vi "Drona Run Tests In Project.vi"   [LabVIEW 2016, in "Script.lvlib"]
uses:
  Script.lvlib
  <vilib>/Wiresmith Technology/G CLI/Argument Parser/Option Class/Option Configuration.ctl
  <vilib>/Wiresmith Technology/G CLI/Argument Parser/Option Class/Argument Type.ctl
  <vilib>/Wiresmith Technology/G CLI/Argument Parser/Option Class/Option.lvclass
  <vilib>/Wiresmith Technology/G CLI/Argument Parser/Option Set Class/Option Set.lvclass
types:
  T1 = typedef "Option Parser.lvlib/Option.lvclass/Option Configuration.ctl" = cluster{"Option Type":T2, "Option Labels":string[], "Key":string, "Description":string, "Required":bool, "Default Value":string}
  T2 = typedef "Option Parser.lvlib/Option.lvclass/Argument Type.ctl" = enum16{"flag", "value"}
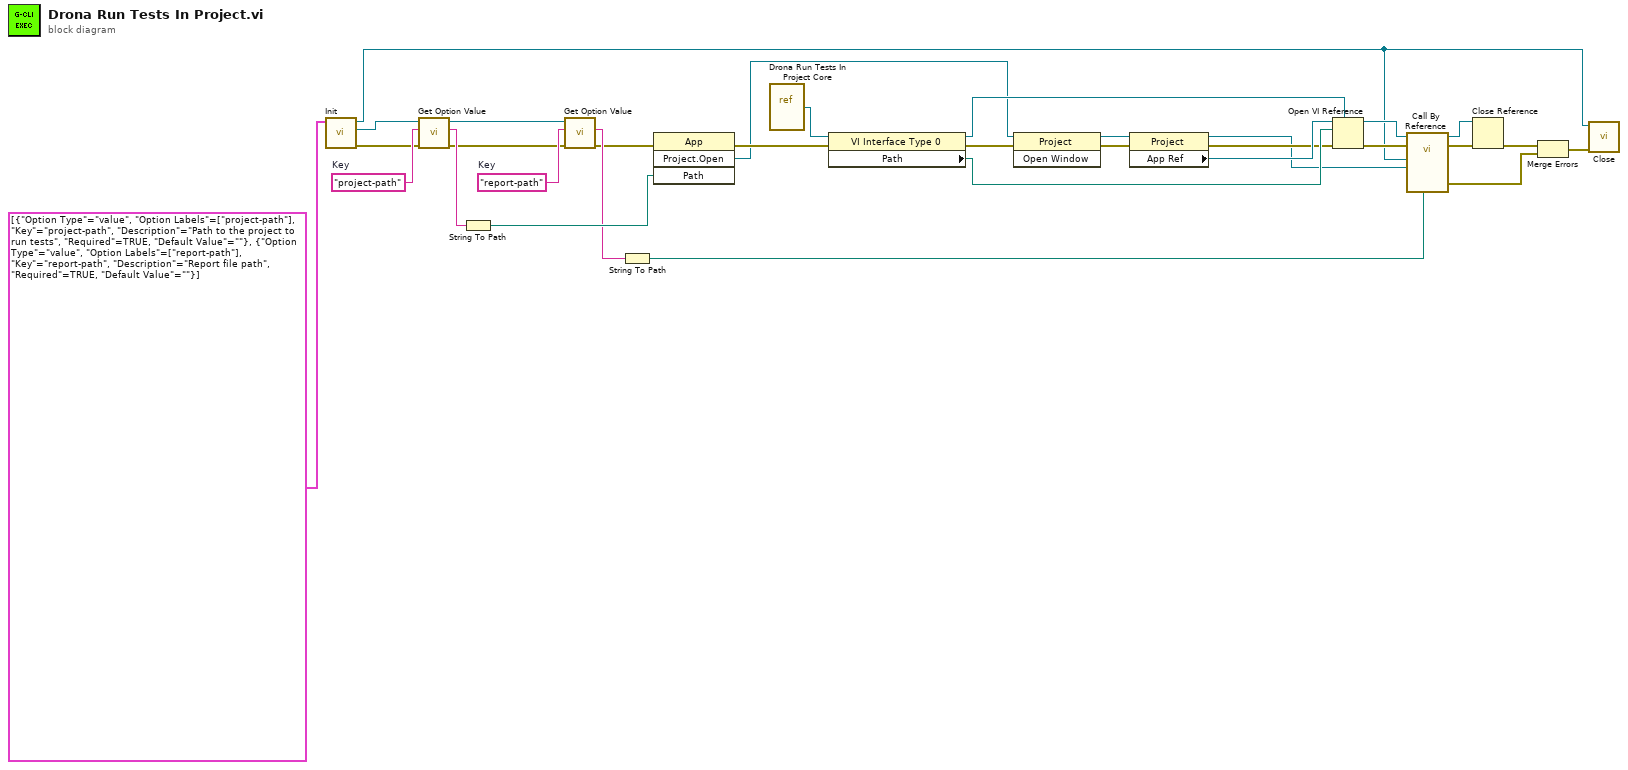
[diagram p0: block diagram]
diagram:
  w14 = "report-path"  # Key
  w19 = "project-path"  # Key
  n1 = call "Init.vi"("Options"=T1[] [{"Option Type"=enum."value", "Option Labels"=["project-path"], "Key"="project-path", "Description"="Path to the project to run tests", "Required"=TRUE, "Default Value"=""}, {"Option Type"=enum."value", "Option Labels"=["report-path"], "Key"="report-path", "Description"="Report file path", "Required"=TRUE, "Default Value"=""}]) -> ("error out"=w18:errorcluster, "Option Set out"=w17:refnum<class "Option Set.lvclass">, "CLI out"=w5:refnum<class "CLI.lvclass">)  [unwired: 8 in]
  n2 = call <vilib>:"Get Option Value.vi"("error in (no error)"=w18, "Option Key"=w19, "Option Set in"=w17) -> ("error out"=w13:errorcluster, "Value"=w16:string, "Option Set out"=w12:refnum<class "Option Set.lvclass">)  [unwired: 5 in, 1 out]
  n3 = String To Path(string=w16) -> (path=w15:path)
  n4 = call <vilib>:"Get Option Value.vi"("error in (no error)"=w13, "Option Key"=w14, "Option Set in"=w12) -> ("error out"=w9:errorcluster, "Value"=w11:string)  [unwired: 5 in, 2 out]
  n5 = String To Path(string=w11) -> (path=w10:path)
  n6 = invoke class="App" method="Project.Open"(error in=w9, "Path"=w15) -> (error out=w8:errorcluster, "Project:Open"=w2:refnum<vi>)  [unwired: 2 in, 2 out]
  n7 = vi-ref "Drona Run Tests In Project Core.vi"() -> (w30:refnum<vi>)
  n8 = property class="VI Interface Type 0"(reference=w30, error in=w8) -> (reference out=w29:refnum<vi>, error out=w4:errorcluster, "Path"=w28:path)
  n9 = invoke class="Project" method="Open Window"(reference=w2, error in=w4) -> (reference out=w1:refnum<vi>, error out=w3:errorcluster)  [unwired: 1 in, 1 out]
  n10 = property class="Project"(reference=w1, error in=w3) -> (reference out=w6:refnum<vi>, error out=w7:errorcluster, "App Ref"=w22:refnum<vi>)
  n11 = Open VI Reference(type specifier VI Refnum (for type only)=w29, application reference (local)=w22, vi path=w28, error in (no error)=w7) -> (vi reference=w26:refnum<vi>, error out=w27:errorcluster)  [unwired: 2 in]
  n12 = call-by-ref "?"(reference=w26, error in=w27, "Report Path"=w10, "Project Reference"=w6, "CLI"=w5) -> (reference out=w24:refnum<vi>, error out=w25:errorcluster, 0:"error out"=w31:errorcluster)  [unwired: 8 in]
  n13 = Close Reference(reference=w24, error in (no error)=w25) -> (error out=w23:errorcluster)
  n14 = Merge Errors(w23, w31) -> (w21:errorcluster)
  n15 = call "Close.vi"("error in (no error)"=w21, "CLI in"=w5) -> ()  [unwired: 10 in]
